vi "Tektronix 7000 Series Width Triggered Acquisition Waveform.vi"() -> ()   [LabVIEW 2015]
doc: "This example VI illustrates how to configure an oscilloscope to generate a width trigger and acquire a waveform from that trigger."
uses:
  <instrlib>/Tektronix 7000 Series/Public/Configure/Configure Trigger (Width).vi
  <instrlib>/Tektronix 7000 Series/Public/Data/Read (Single Waveform).vi
  <instrlib>/Tektronix 7000 Series/Tektronix 7000 Series.lvlib
panel:
  in  "Polarity (0:Positive)":u16(ring) items=["Positive", "Negative"]
  in  "Lower Limit (2E-6s)":dbl=2e-06
  in  "Upper Limit (5E-6s)":dbl=5e-06
  in  "Trigger Condition (1: Outside)":u16(ring)=1 items=["Inside", "Outside"]
  in  "Probe Attenuation (10.0)":dbl=10.0
  in  "Vertical Range (10.0 V)":dbl=10.0
  in  "Timebase (0.005 s)":dbl=0.005
  in  "Vertical Coupling (1: DC)":u16(ring)=1 items=["AC", "DC", "Ground"]
  in  "Channel (0: Channel 1)":u16(ring) format="%#_5f" items=["Channel 1", "Channel 2", "Channel 3", "Channel 4", "Math 1", "Math 2", "Math 3", "Math 4", "Reference 1", "Reference 2", "Reference 3", "Reference 4"]
  in  "VISA Resource Name":refnum<visa-resource-name>
  in  "Trigger Level (0.0)":dbl
  out "Waveform Graph":waveform(dbl)(graph)
  # "(c) 2006 - 2016 National Instruments Corporation.  ALL RIGHTS RESERVED."
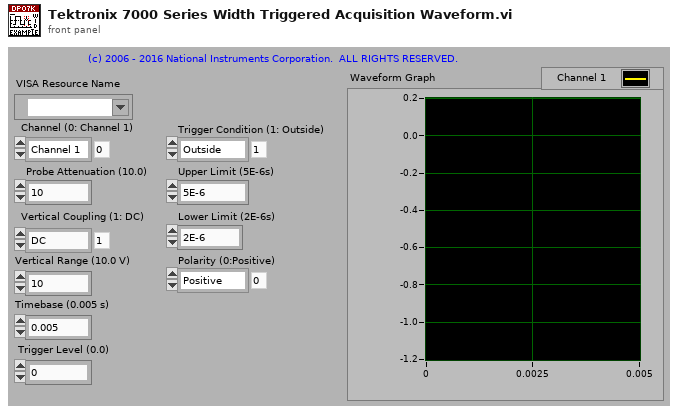
[diagram p1: front panel]
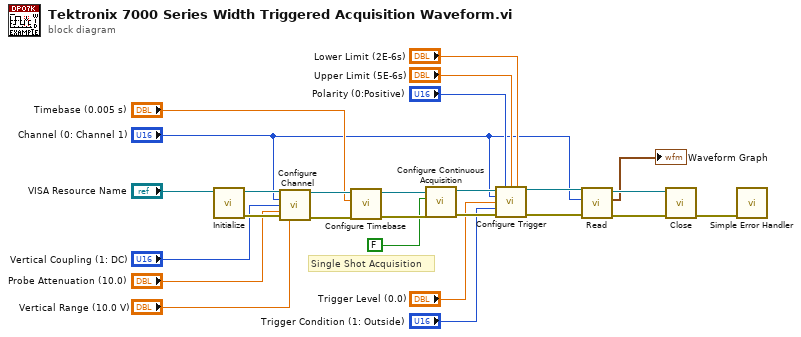
[diagram p0: block diagram]
diagram:
  # "Single Shot Acquisition"
  n1 = call <instrlib>:"Initialize.vi"("VISA resource name"="VISA Resource Name") -> ("error out"=w22:errorcluster, "VISA resource name out"=w23:refnum<visa-resource-name>)  [unwired: 9 in]
  n2 = call <instrlib>:"Configure Channel.vi"("VISA resource name"=w23, "Channel (0: Channel 1)"="Channel (0: Channel 1)", "Vertical Coupling (1: DC)"="Vertical Coupling (1: DC)", "Probe Attenuation (1.0)"="Probe Attenuation (10.0)", "error in (no error)"=w22, "Vertical Range (10.0 V)"="Vertical Range (10.0 V)") -> ("VISA resource name out"=w24:refnum<visa-resource-name>, "error out"=w25:errorcluster)  [unwired: 8 in]
  n3 = call <instrlib>:"Configure Timebase.vi"("error in (no error)"=w25, "Timebase (4 ns)"="Timebase (0.005 s)", "VISA resource name"=w24) -> ("error out"=w20:errorcluster, "VISA resource name out"=w21:refnum<visa-resource-name>)  [unwired: 7 in]
  n4 = call <instrlib>:"Configure Continuous Acquisition.vi"("error in (no error)"=w20, "Enable Continuous Acquisition Mode (True)"=FALSE, "VISA resource name"=w21) -> ("error out"=w17:errorcluster, "VISA resource name out"=w18:refnum<visa-resource-name>)  [unwired: 7 in]
  n5 = call-poly <instrlib>:"Configure Trigger.vi"("VISA resource name"=w18, "Polarity (0:Positive)"="Polarity (0:Positive)", "Upper Limit (5E-6s)"="Upper Limit (5E-6s)", "Lower Limit (2E-6s)"="Lower Limit (2E-6s)", "Source (0:Channel1)"="Channel (0: Channel 1)", "Trigger Level(0V)"="Trigger Level (0.0)", "Trigger Condition (0:Inside)"="Trigger Condition (1: Outside)", "error in (no error)"=w17) -> ("VISA resource name out"=w16:refnum<visa-resource-name>, "error out"=w15:errorcluster)  [unwired: 5 in, 1 out]
  n6 = call-poly <instrlib>:"Read.vi"("error in (no error)"=w15, "Channel (0: Channel 1)"="Channel (0: Channel 1)", "VISA resource name"=w16) -> ("error out"=w12:errorcluster, "Waveform Data"=→"Waveform Graph":waveform(dbl), "VISA resource name out"=w13:refnum<visa-resource-name>)  [unwired: 6 in]
  n7 = call <instrlib>:"Close.vi"("error in (no error)"=w12, "VISA resource name"=w13) -> ("error out"=w14:errorcluster)  [unwired: 9 in]
  n8 = call <vilib>:"Simple Error Handler.vi"("error in (no error)"=w14) -> ()  [unwired: 4 in, 5 out]
